vi "Apply.vi"(8 "error in":errorcluster, 11 "PCAN in":refnum<class "PCAN.lvclass">) -> (0 "error out":errorcluster, 3 "PCAN out":refnum<class "PCAN.lvclass">)   [LabVIEW 2024, in "PCAN.lvclass"]
uses:
  PCAN.lvclass
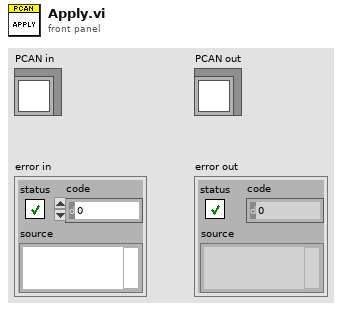
[diagram p1: front panel]
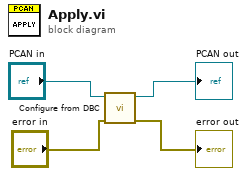
[diagram p0: block diagram]
diagram:
  n1 = call "Configure from DBC.vi"("error in"="error in", "PCAN in"="PCAN in") -> ("error out"=→"error out":errorcluster, "PCAN out"=→"PCAN out":refnum<class "PCAN.lvclass">)  [unwired: 8 in]
